vi "Draw Gradient Write.vi"(4 "error in (no error)":errorcluster, 5 "Value":bool=TRUE, 6 "Container State":T4, 7 "Display State In":T1={"Draw Options"={"Outer Border Color"=0, "Inner Border Color"=6316128, "Outer Gradient Color"=2565927, "Inner Gradient Color"=16860, "Compass North Pointer Color"=16711680, "Compass Pointer Color 1"=13355429, "Compass Pointer Color 2"=14934973, "Direction Pointer Color"=16765184, "Text Box Outline Color"=13355429, "Text Box Background Color"=14934973, "Scale Color"=16448250, "Text Color"=0, "Draw Gradient"=TRUE, "Draw Rose"=TRUE, "Simple Scale"=TRUE, "Draw Text"=FALSE, "Font Name"="Helvetica", "Angle Units"=enum."Degrees"}}) -> (0 "error out":errorcluster, 3 "Display State Out":T1={"Draw Options"={"Outer Border Color"=0, "Inner Border Color"=6316128, "Outer Gradient Color"=2565927, "Inner Gradient Color"=16860, "Compass North Pointer Color"=16711680, "Compass Pointer Color 1"=13355429, "Compass Pointer Color 2"=14934973, "Direction Pointer Color"=16765184, "Text Box Outline Color"=13355429, "Text Box Background Color"=14934973, "Scale Color"=16448250, "Text Color"=0, "Draw Gradient"=TRUE, "Draw Rose"=TRUE, "Simple Scale"=TRUE, "Draw Text"=FALSE, "Font Name"="Helvetica", "Angle Units"=enum."Degrees"}})   [LabVIEW 2017, in "Compass Indicator.xctl"]
uses:
  <vilib>/robotics/Controls/Compass Indicator/Compass Indicator.xctl
  <vilib>/_xctls/Container State.ctl
  <vilib>/robotics/Controls/Compass Indicator/_Compass Indicator Support Files/Compass State.ctl
  <vilib>/robotics/Controls/Compass Indicator/Compass Picture/Draw Options.ctl
  <vilib>/robotics/Controls/Utilities/Angle Units.ctl
  <vilib>/_xctls/XControlSupport.lvlib
  <vilib>/robotics/Controls/Compass Indicator/Compass Picture/NI_Robotics_Compass Picture.lvlib
  <vilib>/robotics/Controls/Utilities/NI_Robotics_Control Utilities.lvlib
panel:
  # "Replace the Value Control below with a Control of desired type.\nDo not remove this Control or the others from the connector pane.\nDo not change the connector pane pattern.\nThe Value control should always be the third terminal from top on the input side in the connector pane."
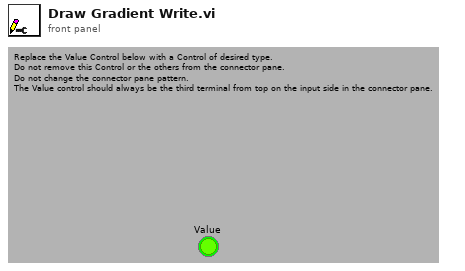
[diagram p1: front panel]
types:
  T1 = typedef "Compass Indicator.xctl/Compass State.ctl" = cluster{"Draw Options":T2}
  T2 = typedef "NI_Robotics_Compass Picture.lvlib/Draw Options.ctl" = cluster{"Outer Border Color":u32, "Inner Border Color":u32, "Outer Gradient Color":u32, "Inner Gradient Color":u32, "Compass North Pointer Color":u32, "Compass Pointer Color 1":u32, "Compass Pointer Color 2":u32, "Direction Pointer Color":u32, "Text Box Outline Color":u32, "Text Box Background Color":u32, "Scale Color":u32, "Text Color":u32, "Draw Gradient":bool, "Draw Rose":bool, "Simple Scale":bool, "Draw Text":bool, "Font Name":string, "Angle Units":T3}
  T3 = typedef "NI_Robotics_Control Utilities.lvlib/Angle Units.ctl" = enum16{"Radians", "Degrees"}
  T4 = typedef "XControlSupport.lvlib/Container State.ctl" = cluster{"Indicator?":bool, "Run Mode?":bool, " Refnum":refnum<vi>}
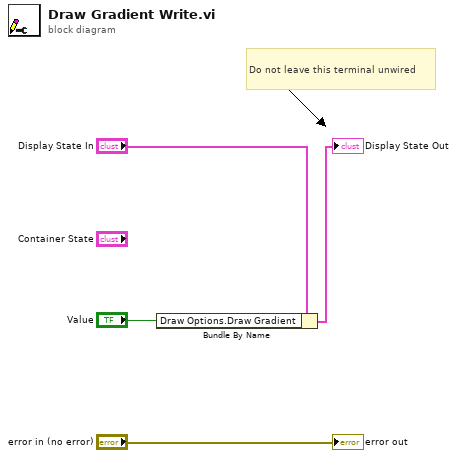
[diagram p0: block diagram]
diagram:
  # "Do not leave this terminal unwired"
  n1 = Bundle By Name(cluster="Display State In", "Draw Options.Draw Gradient"="Value") -> (→"Display State Out":T1)
  "error out" <- "error in (no error)"
